vi "CreateSession.vi"(8 "error in (no error)":errorcluster, 11 "ONNX model path":path) -> (0 "error out":errorcluster, 3 "session id out":i32)   [LabVIEW 2017, in "libonnx_wrapper.lvlib"]
doc: "* @brief Создать новую сессию и загрузить ONNX модель в память\n * \n * Эта функция выделяет уникальный SessionID, загружает модель из файла,\n * анализирует её структуру (входы, выходы, типы данных, формы тензоров)\n * и сохраняет всю информацию для последующего использования.\n * \n * @param modelPath [IN] Путь к файлу модели в формате .onnx (абсолютный или относительный)\n * \n * @return int32: SessionID (положительное целое число >= 1) при успехе\n * @return int32: -1 при ошибке (неверный путь, повреждённая модель, нехватка памяти)\n * \n * @note SessionID необходимо сохранить и передавать во все последующие функции\n * @note При ошибке сессия автоматически удаляется из внутреннего хранилища\n */\nint CreateSession(const char* modelPath);"
uses:
  libonnx_wrapper.lvlib
panel:
  out "wrapper path":path
  out "LastErrorMessage":string
  out "isOk":bool
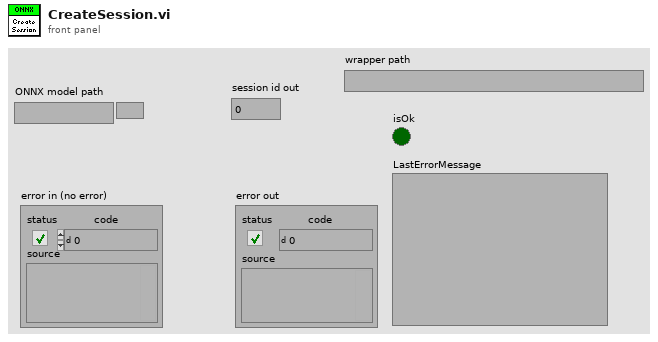
[diagram p1: front panel]
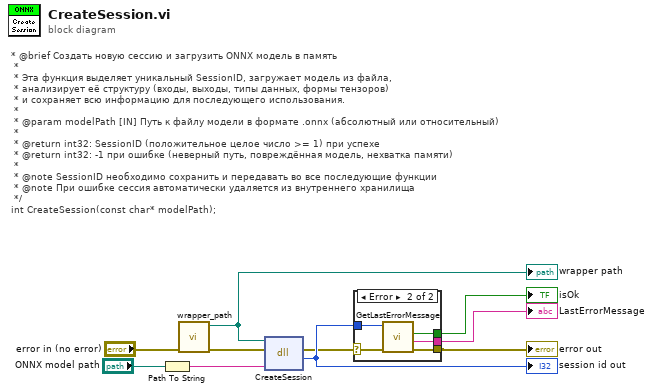
[diagram p0: block diagram]
diagram:
  # "* @brief Создать новую сессию и загрузить ONNX модель в память\n * \n * Эта функция выделяет уникальный SessionID, загружает модель из файла,\n * анализирует её структуру (входы, выходы, типы данных, формы тензоров)\n * и сохраняет всю информацию для последующего использования.\n * \n * @param modelPath [IN] Путь к файлу модели в формате .onnx (абсолютный или относительный)\n * \n * @return int32: SessionID (положительное целое число >= 1) при успехе\n * @return int32: -1 при ошибке (неверный путь, повреждённая модель, нехватка памяти)\n * \n * @note SessionID необходимо сохранить и передавать во все последующие функции\n * @note При ошибке сессия автоматически удаляется из внутреннего хранилища\n */\nint CreateSession(const char* modelPath);"
  n1 = Path To String(path="ONNX model path") -> (string=w9:string)
  n2 = call "wrapper_path.vi"("error in (no error)"="error in (no error)") -> ("error out"=w7:errorcluster, "wrapper path"=w1:path)  [unwired: 9 in]
  "wrapper path" <- w1
  n3 = dll-call lib="home/ivan/LabVIEWData/ONNX/Test/libonnx_wrapper/unix64/libonnx_wrapper.so" fn="CreateSession"(path in=w1, error in=w7, "modelPath"=w9) -> (error out=w5:errorcluster, "return type"=w6:i32)  [unwired: 2 in, 1 out]
  "session id out" <- w6
  n4 = case shown="Error" w5 {
    selector: w5 -> [w11 w15]
    tunnel: w6 -> [_ w16]
    tunnel: [w11 w14] -> w4
    tunnel: [_ w13] -> w3
    tunnel: [_ w12] -> w2
    frame No Error {
    }
    frame Error {
      n5 = call "GetLastErrorMessage.vi"("error in (no error)"=w15, "session id in"=w16) -> ("error out"=w14:errorcluster, "LastErrorMessage"=w12:string, "isOk"=w13:bool)  [unwired: 6 in, 1 out]
    }
  }
  "error out" <- w4
  "isOk" <- w3
  "LastErrorMessage" <- w2
